vi "수신_멀티캐스트2.vi"() -> ()   [LabVIEW 2023]
uses:
  <vilib>/Utility/tcp.llb/UDP Multicast Read-Only Open.vi
panel:
  out "Waveform Graph":dbl[](graph)
  in  "stop":bool
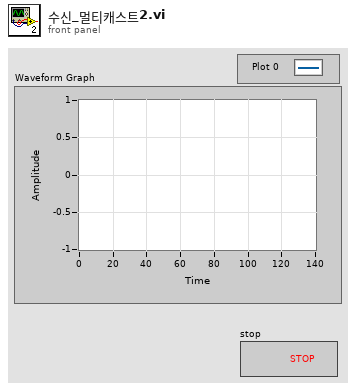
[diagram p1: front panel]
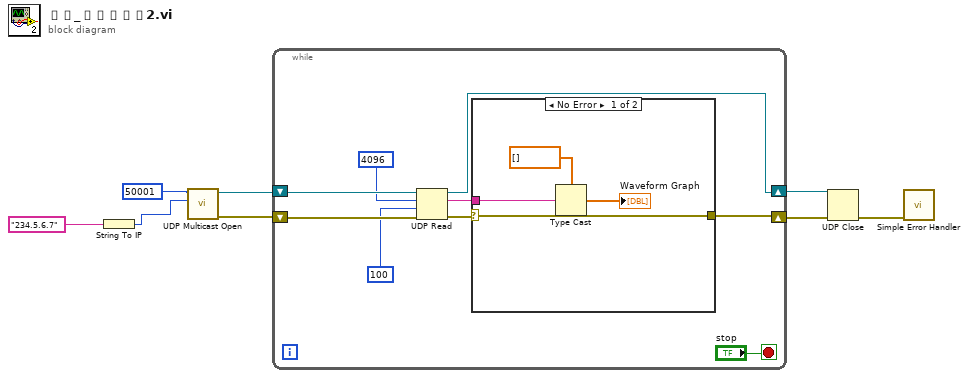
[diagram p0: block diagram]
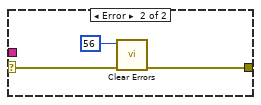
[diagram p2: hidden frame]
diagram:
  n1 = String To IP(1:"234.5.6.7") -> (0:w1:u32)
  n2 = call-poly <vilib>:"UDP Multicast Open.vi"("multicast addr"=w1, "port"=u16 50001) -> ("error out"=w7:errorcluster, "connection ID"=w8:refnum<k16>)  [unwired: 7 in, 1 out]
  n3 = while {
    shift-right: [w16] -> w6
    shift-left: w7 -> [w12]
    shift-right: [w15] -> w4
    shift-left: w8 -> [w14]
    stop <- "stop" stop-if-true
    n4 = UDP Read(connection ID=w14, max size (548)=4096, timeout ms (25000)=100, 8:w12) -> (data out=w13:string, error out=w17:errorcluster, 3:w15:refnum<k16>)  [unwired: 2 out]
    n5 = case shown="No Error" w17 {
      selector: w17 -> [w21 w24]
      tunnel: [w21 w23] -> w16
      tunnel: w13 -> [w20 _]
      frame No Error {
        n6 = Type Cast(type=dbl[] [] ("Waveform Graph"), x=w20) -> (*(type *) &x=→"Waveform Graph":dbl[])
      }
      frame Error {
        n7 = call <vilib>:"Clear Errors.vi"("error in (no error)"=w24, "specific error code to clear (0: all)"=56) -> ("error out"=w23:errorcluster)  [unwired: 4 in, 1 out]
      }
    }
  }
  n8 = UDP Close(connection ID=w4, 8:w6) -> (error out=w5:errorcluster)  [unwired: 1 out]
  n9 = call <vilib>:"Simple Error Handler.vi"("error in (no error)"=w5) -> ()  [unwired: 4 in, 5 out]
